vi "Test Get Output.vi"() -> ()   [LabVIEW 2016, in "Spectrum Recorder too.lvclass"]
uses:
  Spectrum Recorder too.lvclass
  Spectrum Recorder too.lvclass/Spectrum Recorder too.ctl
  Read Spectrum Recorder Configuration.vi
  Write Spectrum Recorder Configuration.vi
panel:
  out "size(s)":i32
  out "Output values out":dbl[](array[numeric])
  out "Waveform Graph":dbl[](graph)
  in  "Number of points":i32=100
  in  "User Configuration.Repeat (-1: forever)":i32=1
  in  "Output counter":i32
  in  "Records counter":i32
  in  "Output values in":dbl[](array[numeric])=[1.0, 2.0, 3.0, 4.0, 5.0, 6.0, 7.0, 8.0, 9.0, 10.0]
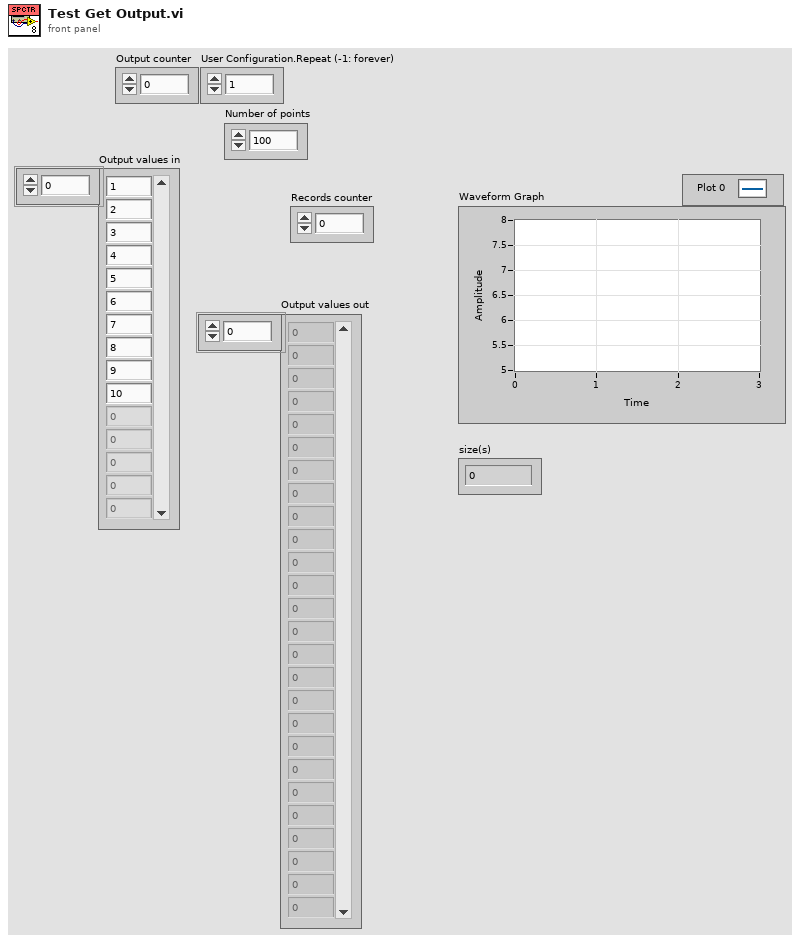
[diagram p1: front panel]
types:
  T1 = typedef "Spectrum Recorder Configuration.ctl" = cluster{"Start":dbl, "End":dbl, "Duration":dbl, "Filter time constant":dbl, "Repeat (-1: forever)":i32, "Update rate":dbl, "Data storage folder":path}
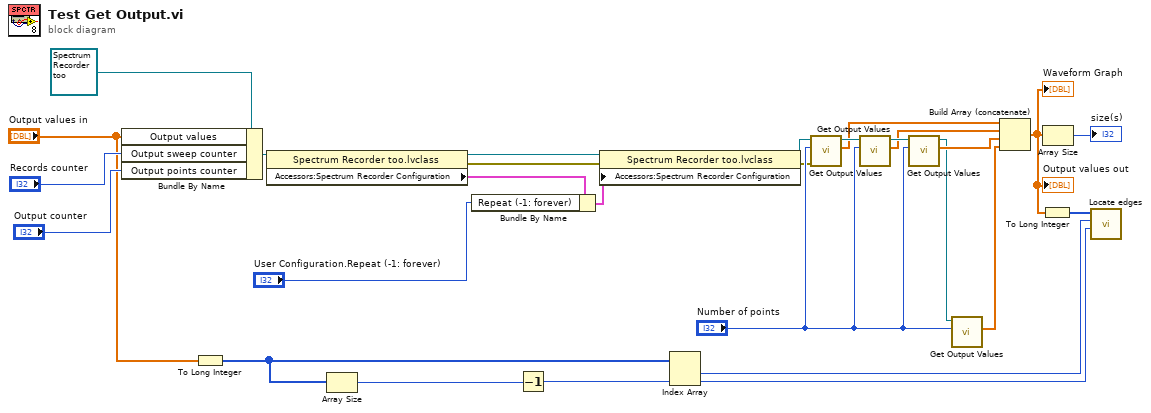
[diagram p0: block diagram]
diagram:
  n1 = Bundle By Name(cluster=refnum<class "Spectrum Recorder too.lvclass"> refnum ("Spectrum Recorder.lvclass"), "Output values"="Output values in", "Output sweep counter"="Records counter", "Output points counter"="Output counter") -> (w25:refnum<class "Spectrum Recorder too.lvclass">)
  n2 = To Long Integer(number="Output values in") -> (32bit integer=w9:i32[])
  n3 = property class="Spectrum Recorder too.lvclass"(reference=w25) -> (reference out=w5:refnum<class "Spectrum Recorder too.lvclass">, error out=w2:errorcluster, "Accessors:Spectrum Recorder Configuration"=w7:T1)  [unwired: 1 in]
  n4 = Array Size(array=w9) -> (size(s)=w14:i32)
  n5 = Bundle By Name(cluster=w7, "Repeat (-1: forever)"="User Configuration.Repeat (-1: forever)") -> (w6:T1)
  n6 = Decrement(x=w14) -> (x-1=w13:i32)
  n7 = property class="Spectrum Recorder too.lvclass"(reference=w5, error in=w2, "Accessors:Spectrum Recorder Configuration"=w6) -> (reference out=w4:refnum<class "Spectrum Recorder too.lvclass">, error out=w3:errorcluster)
  n8 = Index Array(array=w9, index #2=w13) -> (element #1=w12:i32, element #2=w11:i32)  [unwired: 1 in]
  n9 = call-dynamic "Get Output Values.vi"("error in (no error)"=w3, "Number of points"="Number of points", "Spectrum Recorder in"=w4) -> ("Output values"=w21:dbl[], "Spectrum Recorder out"=w23:refnum<class "Spectrum Recorder too.lvclass">)  [unwired: 6 in, 1 out]
  n10 = call-dynamic "Get Output Values.vi"("Number of points"="Number of points", "Spectrum Recorder in"=w23) -> ("Output values"=w20:dbl[], "Spectrum Recorder out"=w22:refnum<class "Spectrum Recorder too.lvclass">)  [unwired: 7 in, 1 out]
  n11 = call-dynamic "Get Output Values.vi"("Number of points"="Number of points", "Spectrum Recorder in"=w22) -> ("Output values"=w19:dbl[], "Spectrum Recorder out"=w18:refnum<class "Spectrum Recorder too.lvclass">)  [unwired: 7 in, 1 out]
  n12 = call-dynamic "Get Output Values.vi"("Number of points"="Number of points", "Spectrum Recorder in"=w18) -> ("Output values"=w16:dbl[])  [unwired: 7 in, 2 out]
  n13 = Build Array (concatenate)(w21, w20, w19, w16) -> (w15:dbl[])
  "Waveform Graph" <- w15
  "Output values out" <- w15
  n14 = To Long Integer(number=w15) -> (32bit integer=w8:i32[])
  n15 = Array Size(array=w15) -> (size(s)=→"size(s)":i32)
  n16 = call "Locate edges.vi"("Last value"=w11, "First value"=w12, "Values"=w8) -> ()  [unwired: 7 in, 2 out]
